vi "Periodic Tasks.vi"(8 "error in":errorcluster) -> ()   [LabVIEW 2017]
doc: "This VI runs in parallel to other tasks. It can contain as many user-defined periodic loops as you need. These can carry out PID or other sorts of timed response."
uses:
  <vilib>/Rock Robotics/WPI/ThirdParty/Phoenix-LabVIEW/Motor Controller/Controls/CTRE_Phoenix_MotorControl_FeedbackDevice.ctl
  <vilib>/Rock Robotics/WPI/Utilities/WPI_GetSetVariantRefNum.vi
  <vilib>/Rock Robotics/Network Tables/NT Write Numeric Array.vi
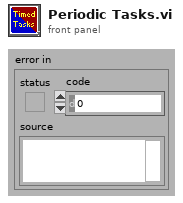
[diagram p1: front panel]
types:
  T1 = cluster{"Yaw":dbl, "Roll":dbl, "Pitch":dbl, "Heading":dbl, "Fused Heading":dbl}
  T2 = typedef "WPI_JoystickDevRef.ctl" = cluster{"Device":T3}
  T3 = typedef "WPI_JoystickDeviceEnum.ctl" = enum16{"USB 0", "USB 1", "USB 2", "USB 3", "USB 4", "USB 5"}
  T4 = cluster{"Motor1":cluster{"P":dbl, "I":dbl, "D":dbl}, "Motor3":cluster{"P":dbl, "I":dbl, "D":dbl}, "Motor2":cluster{"P":dbl, "I":dbl, "D":dbl}, "Motor4":cluster{"P":dbl, "I":dbl, "D":dbl}}
  T5 = cluster{"Buttons[0]":bool, "Buttons[1]":bool, "Buttons[2]":bool, "Buttons[3]":bool, "Buttons[4]":bool, "Buttons[5]":bool, "Buttons[6]":bool, "Buttons[7]":bool, "Buttons[8]":bool}
  T6 = typedef "CTRE_Phoenix_MotorControl_FeedbackDevice.ctl" = i8
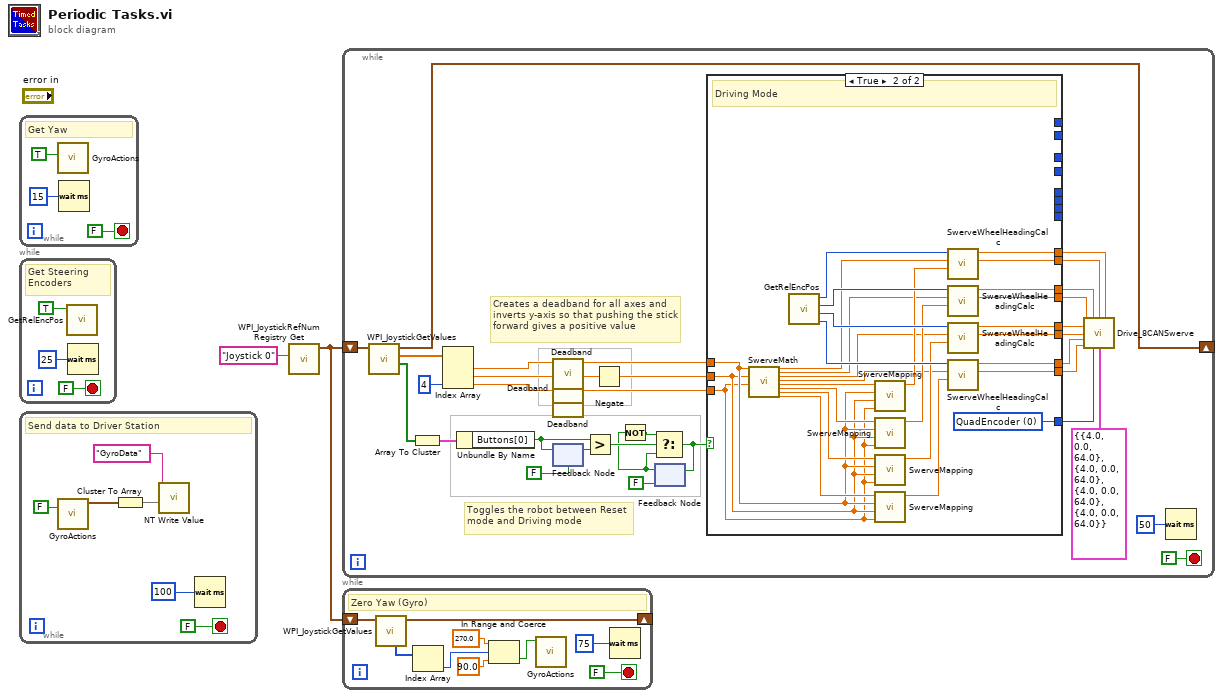
[diagram p0: block diagram]
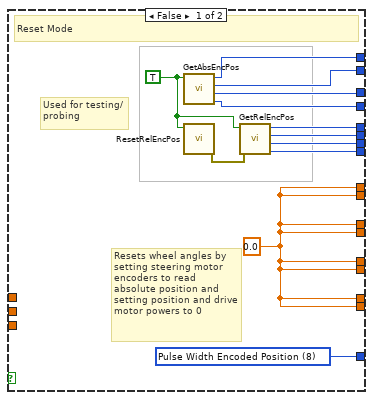
[diagram p2: hidden frame]
diagram:
  n1 = while {
    stop <- FALSE stop-if-true
    # "Get Yaw"
    n2 = call "GyroActions.vi"("Update?"=TRUE ("Zero")) -> ()  [unwired: 9 in, 2 out]
    n3 = Wait (ms)(milliseconds to wait=u32 15) -> ()  [unwired: 1 out]
  }
  n4 = while {
    stop <- FALSE stop-if-true
    # "Get Steering Encoders"
    n5 = call "GetRelEncPos.vi"("Update?"=TRUE ("Zero")) -> ()  [unwired: 6 in, 5 out]
    n6 = Wait (ms)(milliseconds to wait=u32 25) -> ()  [unwired: 1 out]
  }
  n7 = while {
    stop <- FALSE stop-if-true
    # "Send data to Driver Station"
    n8 = call "GyroActions.vi"("Zero"=FALSE) -> ("YRPHfH"=w12:T1)  [unwired: 9 in, 1 out]
    n9 = Cluster To Array(cluster=w12) -> (array=w11:dbl[])
    n10 = call-poly <vilib>:"NT Write Value.vi"("Numeric Array"=w11, "Name"="GyroData") -> ()  [unwired: 9 in, 1 out]
    n11 = Wait (ms)(milliseconds to wait=u32 100 ("millisecond timer value")) -> ()  [unwired: 1 out]
  }
  n12 = call <vilib>:"WPI_JoystickRefNum Registry Get.vi"("refnum name"="Joystick 0") -> ("JoystickDevRef"=w1:T2)  [unwired: 1 in, 9 out]
  n13 = while {
    shift-right: [w45] -> _
    shift-left: w1 -> [w46]
    stop <- FALSE stop-if-true
    # "Creates a deadband for all axes and inverts y-axis so that pushing the stick forward gives a positive value"
    # "Toggles the robot between Reset mode and Driving mode"
    n14 = call <vilib>:"WPI_JoystickGetValues.vi"("JoystickDevRef"=w46) -> ("Buttons"=w34:bool[], "Axes"=w36:dbl[], "JoystickDevRef"=w45:T2)  [unwired: 6 in, 2 out]
    n15 = Array To Cluster(array=w34) -> (cluster=w33:T5)
    n16 = Index Array(array=w36, index #3=4 ("index")) -> (element #1=w22:dbl, element #2=w23:dbl, element #3=w24:dbl)  [unwired: 2 in]
    n17 = Unbundle By Name(w33) -> ("Buttons[0]"=w29:bool)
    n18 = call "Deadband.vi"("Input"=w22) -> ("Output"=w21:dbl)  [unwired: 6 in]
    n19 = call "Deadband.vi"("Input"=w23) -> ("Output"=w18:dbl)  [unwired: 6 in]
    n20 = call "Deadband.vi"("Input"=w24) -> ("Output"=w20:dbl)  [unwired: 6 in]
    n21 = feedback #1(FALSE) -> (w30:bool)
    n22 = feedback-in #1(w29) -> ()
    n23 = Greater?(x=w29, y=w30) -> (0:w31:bool)
    n24 = Negate(x=w18) -> (-x=w17:dbl)
    n25 = feedback #2(FALSE) -> (w27:bool)
    n26 = Not(x=w27) -> (.not. x?=w26:bool)
    n27 = Select(t=w26, s=w31, f=w27) -> (s? t:f=w25:bool)
    n28 = feedback-in #2(w25) -> ()
    n29 = case shown="True" w25 {
      tunnel: w21 -> [_ w66]
      tunnel: w17 -> [_ w65]
      tunnel: [w48 w83] -> w37
      tunnel: [w48 w76] -> w19
      tunnel: [w48 w81] -> w42
      tunnel: [w48 w82] -> w43
      tunnel: [w48 w87] -> w38
      tunnel: [w48 w86] -> w39
      tunnel: [w48 w85] -> w40
      tunnel: [w48 w84] -> w41
      tunnel: w20 -> [_ w64]
      tunnel: [w59 _] -> _
      tunnel: [w58 _] -> _
      tunnel: [w57 _] -> _
      tunnel: [w56 _] -> _
      tunnel: [w55 w77] -> w16
      tunnel: [w52 _] -> _
      tunnel: [w51 _] -> _
      tunnel: [w50 _] -> _
      tunnel: [w49 _] -> _
      frame False {
        w55 = T6 8 items=["None"=-1, "QuadEncoder"=0, "Analog"=2, "Tachometer"=4, "Pulse Width Encoded Position"=8, "Sensor Sum (S0 + S1)"=9, "Sensor Difference (D0 - D1)"=10, "Remote Source 0"=11, "Remote Source 1"=12, "Software Emulated"=15] ("Feedback Device")
        w53 = TRUE ("Update?")
        w48 = 0.0 ("P")
        # "Resets wheel angles by setting steering motor encoders to read absolute position and setting position and drive motor powers to 0"
        # "Used for testing/probing"
        # "Reset Mode"
        n30 = call "GetAbsEncPos.vi"("Update?"=w53) -> ("RearRightPulsePos"=w56:i32, "RearLeftPulsePos"=w57:i32, "FrontRightPulsePos"=w58:i32, "FrontLeftPulsePos"=w59:i32)  [unwired: 7 in]
        n31 = call "GetRelEncPos.vi"("Update?"=w53) -> ("RearRightQuadPos"=w49:i32, "RearLeftQuadPos"=w50:i32, "FrontRightQuadPos"=w51:i32, "FrontLeftQuadPos"=w52:i32, "error in"=w54:errorcluster)  [unwired: 6 in]
        n32 = call "ResetRelEncPos.vi"("error in"=w54, "Reset?"=w53) -> ()  [unwired: 10 in]
      }
      frame True {
        w77 = T6 0 items=["None"=-1, "QuadEncoder"=0, "Analog"=2, "Tachometer"=4, "Pulse Width Encoded Position"=8, "Sensor Sum (S0 + S1)"=9, "Sensor Difference (D0 - D1)"=10, "Remote Source 0"=11, "Remote Source 1"=12, "Software Emulated"=15] ("Feedback Device")
        # "Driving Mode"
        n33 = call "SwerveMath.vi"("X-Axis"=w66, "Y-Axis"=w65, "Turn"=w64) -> ("FrontLeftTarget"=w60:dbl, "FrontRightTarget"=w61:dbl, "RearLeftTarget"=w62:dbl, "RearRightTarget"=w63:dbl, "FrontLeftDrive"=w70:dbl, "FrontRightDrive"=w69:dbl, "RearLeftDrive"=w68:dbl, "RearRightDrive"=w67:dbl)  [unwired: 17 in]
        n34 = call "GetRelEncPos.vi"() -> ("RearRightQuadPos"=w79:i32, "RearLeftQuadPos"=w78:i32, "FrontRightQuadPos"=w80:i32, "FrontLeftQuadPos"=w75:i32)  [unwired: 7 in, 1 out]
        n35 = call "SwerveMapping.vi"("Turn"=w64, "Y Axis"=w65, "X Axis"=w66, "DriveIn"=w70) -> ("DriveOut"=w74:dbl)  [unwired: 7 in]
        n36 = call "SwerveMapping.vi"("Turn"=w64, "Y Axis"=w65, "X Axis"=w66, "DriveIn"=w69) -> ("DriveOut"=w73:dbl)  [unwired: 7 in]
        n37 = call "SwerveMapping.vi"("Turn"=w64, "Y Axis"=w65, "X Axis"=w66, "DriveIn"=w68) -> ("DriveOut"=w72:dbl)  [unwired: 7 in]
        n38 = call "SwerveMapping.vi"("Turn"=w64, "Y Axis"=w65, "X Axis"=w66, "DriveIn"=w67) -> ("DriveOut"=w71:dbl)  [unwired: 7 in]
        n39 = call "SwerveWheelHeadingCalc.vi"("DriveIn"=w74, "Target"=w60, "Current"=w75) -> ("DriveOut"=w81:dbl, "TargetFinal"=w76:dbl)  [unwired: 7 in]
        n40 = call "SwerveWheelHeadingCalc.vi"("DriveIn"=w73, "Target"=w61, "Current"=w80) -> ("DriveOut"=w83:dbl, "TargetFinal"=w82:dbl)  [unwired: 7 in]
        n41 = call "SwerveWheelHeadingCalc.vi"("DriveIn"=w72, "Target"=w62, "Current"=w78) -> ("DriveOut"=w85:dbl, "TargetFinal"=w84:dbl)  [unwired: 7 in]
        n42 = call "SwerveWheelHeadingCalc.vi"("DriveIn"=w71, "Target"=w63, "Current"=w79) -> ("DriveOut"=w87:dbl, "TargetFinal"=w86:dbl)  [unwired: 7 in]
      }
    }
    n43 = call "Drive_8CANSwerve.vi"("FrontRightDrive"=w37, "FrontRightRotation"=w43, "FrontLeftDrive"=w42, "FrontLeftRotation"=w19, "RearLeftRotation"=w41, "RearLeftDrive"=w40, "RearRightRotation"=w39, "RearRightDrive"=w38, "Feedback Device"=w16, "PIDInputs"=T4 {"Motor1"={"P"=4.0, "I"=0.0, "D"=64.0}, "Motor3"={"P"=4.0, "I"=0.0, "D"=64.0}, "Motor2"={"P"=4.0, "I"=0.0, "D"=64.0}, "Motor4"={"P"=4.0, "I"=0.0, "D"=64.0}}) -> ()  [unwired: 6 in]
    n44 = Wait (ms)(milliseconds to wait=u32 50) -> ()  [unwired: 1 out]
  }
  n45 = while {
    shift-right: [w89] -> _
    shift-left: w1 -> [w96]
    stop <- FALSE stop-if-true
    # "Zero Yaw (Gyro)"
    n46 = call <vilib>:"WPI_JoystickGetValues.vi"("JoystickDevRef"=w96) -> ("JoystickDevRef"=w89:T2, "POVs"=w94:i16[])  [unwired: 6 in, 3 out]
    n47 = Index Array(array=w94) -> (element=w93:i16)  [unwired: 1 in]
    n48 = In Range and Coerce(upper limit=270.0, x=w93, lower limit=90.0) -> (In Range?=w92:bool)  [unwired: 1 out]
    n49 = call "GyroActions.vi"("Zero"=w92) -> ()  [unwired: 9 in, 2 out]
    n50 = Wait (ms)(milliseconds to wait=u32 75) -> ()  [unwired: 1 out]
  }
